vi "main.vi"(0 "TDMS File Path":path, 11 "Error In":errorcluster) -> (15 "Error Out":errorcluster)   [LabVIEW 2023]
uses:
  <vilib>/Utility/NIReport.llb/Report Type.ctl
  <vilib>/SLL Toolkit/SLL String/_SubVIs/I32 to String.vi
  <vilib>/Utility/NIReport.llb/NI_report.lvclass
  <vilib>/Utility/NIReport.llb/NI_ReportGenerationCore.lvlib
  <vilib>/Utility/NIReport.llb/Excel/NI_Excel.lvclass
  <vilib>/SLL Toolkit/SLL String/SLL String.lvlib
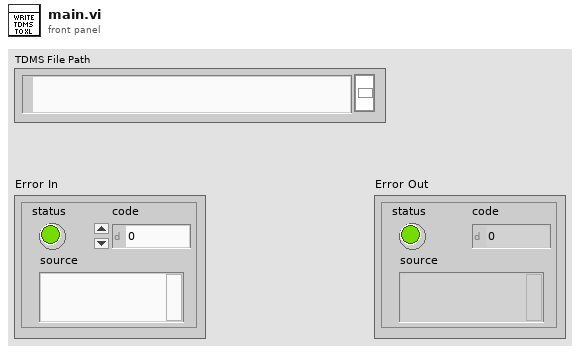
[diagram p1: front panel]
types:
  T1 = typedef "NI_ReportGenerationCore.lvlib/Report Type.ctl" = enum16{"HTML", "Word", "Excel"}
  T2 = enum16{"open", "open or create", "create or replace", "create", "open (read-only)"}
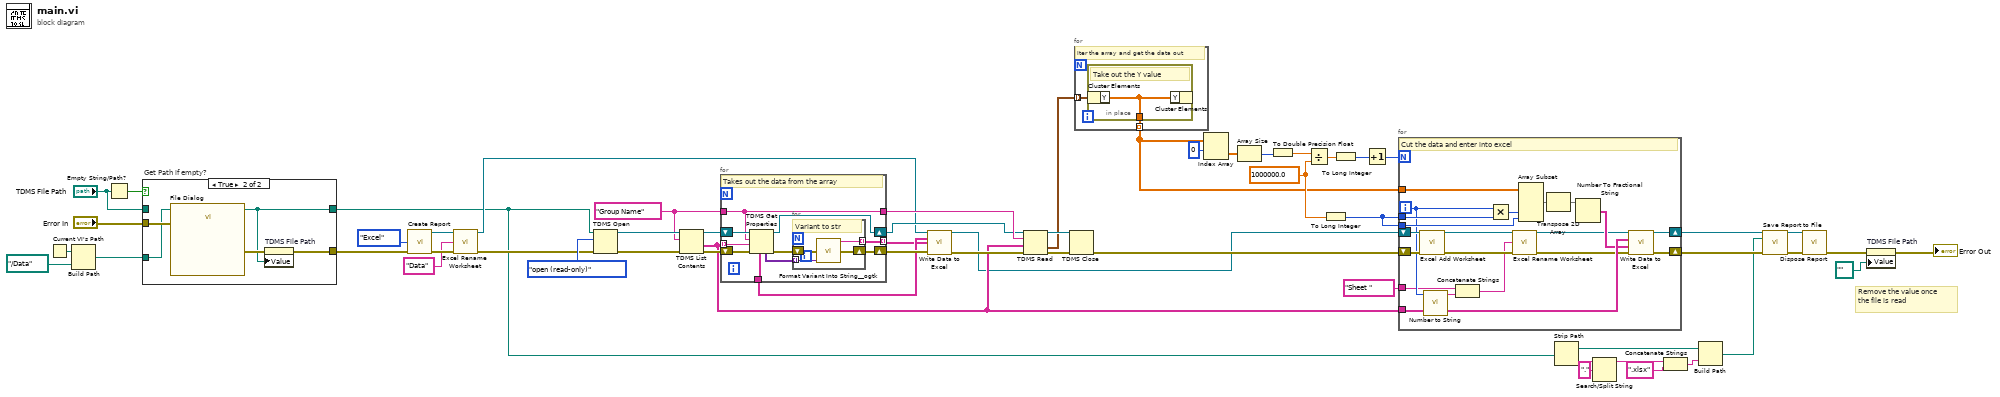
[diagram p0: block diagram]
diagram:
  w31 = 1000000.0 ("y")
  w47 = "Group Name"
  # "Remove the value once the file is read"
  n1 = Current VI's Path() -> (path=w46:path)
  n2 = Build Path(base path=w46, name or relative path=path "../Data") -> (appended path=w44:path)
  n3 = Empty String/Path?(string/path="TDMS File Path") -> (empty?=w56:bool)
  n4 = case "Get Path if empty?" shown="True" w56 {
    tunnel: "Error In" -> [w59 w64]
    tunnel: [w59 w62] -> w53
    tunnel: "TDMS File Path" -> [w58 _]
    tunnel: [w58 w61] -> w13
    tunnel: w44 -> [_ w60]
    frame False {
    }
    frame True {
      n5 = call "File Dialog"("start path"=w60, "error in"=w64) -> ("selected path"=w61:path, "error out"=w63:errorcluster)  [unwired: 10 in, 2 out]
      n6 = property on="TDMS File Path" class="Path"(error in=w63, "Value"=w61) -> (error out=w62:errorcluster)  [unwired: 1 in, 1 out]
    }
  }
  n7 = call <vilib>:"Create Report.vi"("report type"=Report_Type."Excel", "error in (no error)"=w53) -> ("report out"=w19:refnum<class "NI_report.lvclass">, "error out"=w24:errorcluster)  [unwired: 12 in]
  n8 = call <vilib>:"Excel Rename Worksheet.vi"("report in"=w19, "worksheet name (\"\")"="Data", "error in (no error)"=w24) -> ("report out"=w18:refnum<class "NI_report.lvclass">, "error out"=w20:errorcluster)  [unwired: 11 in]
  n9 = TDMS Open(8:w20, 10:T2."open (read-only)" ("operation (0:open)"), 11:w13) -> (0:w52:errorcluster, 3:w49:refnum<k34>)  [unwired: 4 in]
  n10 = TDMS List Contents(4:w52, 6:w47, 7:w49) -> (0:w50:errorcluster, 1:w27:string[], 3:w48:refnum<k34>)  [unwired: 1 out]
  n11 = for {
    tunnel: w47 -> [w65]
    shift-right: [w68] -> w51
    shift-left: w50 -> [w72]
    shift-right: [w73] -> w38
    shift-left: w48 -> [w71]
    tunnel: w27 -> [w70] mode=indexing
    tunnel: [w69] -> w23
    tunnel: [w66] -> w22 mode=indexing
    tunnel: [w65] -> w39
    # "Takes out the data from the array"
    n12 = TDMS Get Properties(8:w72, 9:w70, 10:w65, 11:w71) -> (0:w74:errorcluster, 3:w73:refnum<k34>, 4:w67:variant[], 6:w69:string[])  [unwired: 2 in, 2 out]
    n13 = for {
      tunnel: w67 -> [w76] mode=indexing
      shift-right: [w77] -> w68
      shift-left: w74 -> [w78]
      tunnel: [w75] -> w66 mode=indexing
      # "Variant to str"
      n14 = call <userlib>:"Format Variant Into String__ogtk.vi"("error in (no error)"=w78, "Variant"=w76) -> ("Output String"=w75:string, "error out"=w77:errorcluster)  [unwired: 12 in]
    }
  }
  n15 = call "Write Data to Excel.vi"("Report In"=w18, "Header Array"=w23, "Data Array"=w22, "Error In"=w51) -> ("Report Out"=w21:refnum<class "NI_report.lvclass">, "Error Out"=w43:errorcluster)  [unwired: 10 in]
  n16 = TDMS Read(0:w38, 5:w39, 7:w27, 11:w43) -> (4:w41:refnum<k34>, 10:w36:waveform(dbl)[], 15:w40:errorcluster)  [unwired: 4 in, 3 out]
  n17 = TDMS Close(8:w40, 11:w41) -> (0:w28:errorcluster)  [unwired: 1 out]
  n18 = for {
    tunnel: w36 -> [w80] mode=indexing
    tunnel: [w79] -> w30 mode=indexing
    # "Iter the array and get the data out"
    n19 = in-place {
      in-place-border: [w81] -> w79
      # "Take out the Y value"
      n20 = in-place-cluster #1(w80) -> ("Y"=w81:dbl[])
      n21 = in-place-cluster #1("Y"=w81) -> ()  [unwired: 1 out]
    }
  }
  n22 = Index Array(array=w30, index (row)=0) -> (element=w34:dbl[])  [unwired: 1 in]
  n23 = Array Size(array=w34) -> (size(s)=w33:i32)
  n24 = To Double Precision Float(number=w33) -> (double precision float=w32:dbl)
  n25 = Divide(x=w32, y=w31) -> (x/y=w2:dbl)
  n26 = To Long Integer(number=w31) -> (32bit integer=w29:i32)
  n27 = To Long Integer(number=w2) -> (32bit integer=w3:i32)
  n28 = Increment(x=w3) -> (x+1=w1:i32)
  n29 = for {
    N: w1 -> [_]
    tunnel: w29 -> [w101]
    tunnel: w30 -> [w100]
    tunnel: w29 -> [w98]
    shift-right: [w93] -> w26
    shift-left: w28 -> [w90]
    tunnel: w27 -> [w96]
    shift-right: [w92] -> w14
    shift-left: w21 -> [w91]
    tunnel: "Sheet " -> [w84]
    i -> [w85]
    # "Cut the data and enter into excel"
    n30 = call <vilib>:"Excel Add Worksheet.vi"("report in"=w91, "error in (no error)"=w90) -> ("report out"=w87:refnum<class "NI_report.lvclass">, "error out"=w89:errorcluster)  [unwired: 12 in]
    n31 = call-poly <vilib>:"Number to String.vi"("Numeric"=w85) -> ("String"=w83:string)  [unwired: 10 in]
    n32 = Concatenate Strings(w84, w83) -> (w82:string)
    n33 = Multiply(x=w85, y=w101) -> (x*y=w99:i32)
    n34 = call <vilib>:"Excel Rename Worksheet.vi"("report in"=w87, "worksheet name (\"\")"=w82, "error in (no error)"=w89) -> ("report out"=w86:refnum<class "NI_report.lvclass">, "error out"=w88:errorcluster)  [unwired: 11 in]
    n35 = Array Subset(array=w100, index (col)=w99, length (col)=w98) -> (w97:dbl[][])  [unwired: 2 in]
    n36 = Transpose 2D Array(2D array=w97) -> (transposed array=w94:dbl[][])
    n37 = Number To Fractional String(number=w94) -> (F-format string=w95:string[][])  [unwired: 3 in]
    n38 = call "Write Data to Excel.vi"("Report In"=w86, "Header Array"=w96, "Data Array"=w95, "Error In"=w88) -> ("Report Out"=w92:refnum<class "NI_report.lvclass">, "Error Out"=w93:errorcluster)  [unwired: 10 in]
  }
  n39 = Strip Path(path=w13) -> (stripped path=w7:path, name=w12:string)
  n40 = Search/Split String(string=w12, search string/char (-)=".") -> (substring before match=w10:string)  [unwired: 1 in, 2 out]
  n41 = Concatenate Strings(w10, ".xlsx" ("string")) -> (w8:string)
  n42 = Build Path(base path=w7, name or relative path=w8) -> (appended path=w6:path)
  n43 = call-dynamic "Save Report to File.vi"("report in"=w14, "report file path"=w6, "error in (no error)"=w26) -> ("report out"=w4:refnum<class "NI_report.lvclass">, "error out"=w15:errorcluster)  [unwired: 11 in]
  n44 = call-dynamic "Dispose Report.vi"("report in"=w4, "error in (no error)"=w15) -> ("error out"=w5:errorcluster)  [unwired: 13 in]
  n45 = property on="TDMS File Path" class="Path"(error in=w5, "Value"=path "" ("TDMS File Path")) -> (error out=→"Error Out":errorcluster)  [unwired: 1 in, 1 out]
